vi "Serial Port Read.vi"(7 "stop":bool, 8 "error in (no error)":errorcluster, 9 "Timeout (2000ms)":u32=2000, 10 "Byte Count":u32, 11 "VISA resource name":refnum<visa-resource-name>) -> (0 "error out":errorcluster, 1 "Return Count":u32, 2 "Read Buffer":string, 3 "VISA resource name out":refnum<visa-resource-name>)   [LabVIEW 2009, in "DSO1K.lvlib"]
doc: "Serial port that you set for this vi."
uses:
  <instrlib>/DSO1K/DSO1K.lvlib
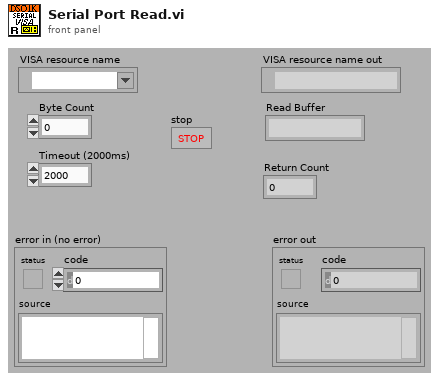
[diagram p1: front panel]
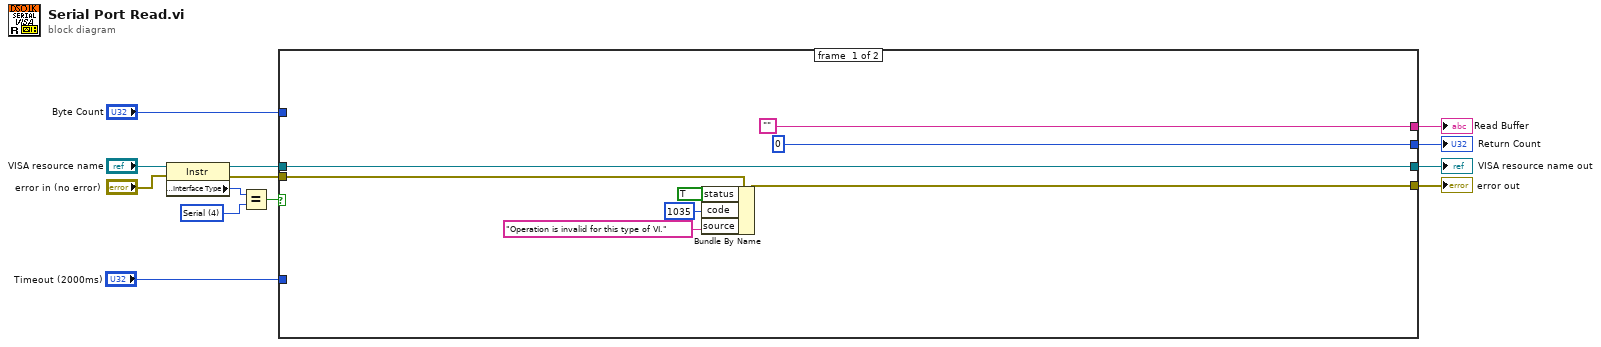
[diagram p0: block diagram]
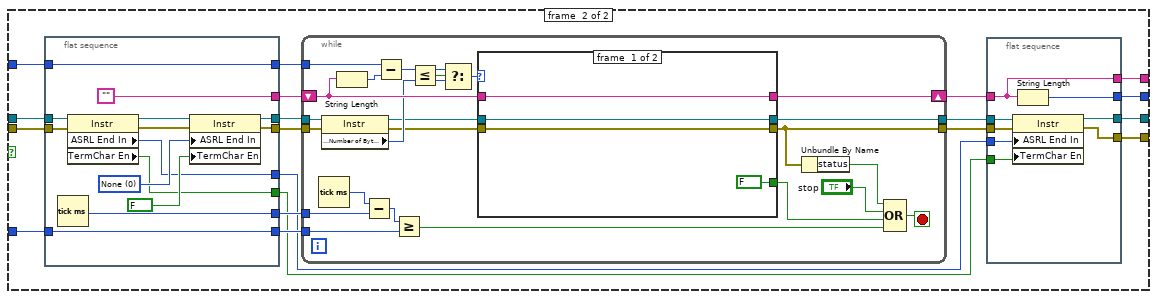
[diagram p2: hidden frame]
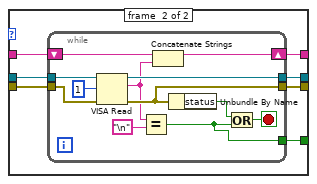
[diagram p3: hidden frame]
diagram:
  w3 = u16 4 items=["GPIB"=1, "VXI"=2, "GPIB-VXI"=3, "Serial"=4, "PXI"=5, "TCPIP"=6, "USB"=7, "FireWire"=9] ("Interface Information:Interface Type")
  n1 = property class="Instr"(reference="VISA resource name", error in="error in (no error)") -> (reference out=w13:refnum<visa-resource-name>, error out=w12:errorcluster, "Interface Information:Interface Type"=w4:u16)
  n2 = Equal?(x=w4, y=w3) -> (x = y?=w2:bool)
  n3 = case shown="True" w2 {
    tunnel: w13 -> [w19 w36]
    tunnel: w12 -> [w18 w35]
    tunnel: ["" w24] -> w6
    tunnel: [w19 w25] -> w9
    tunnel: [w17 w28] -> w8
    tunnel: [u32 0 ("return count") w30] -> w10
    tunnel: "Byte Count" -> [_ w32]
    tunnel: "Timeout (2000ms)" -> [_ w31]
    frame #0 {
      n4 = Bundle By Name(cluster=w18, "status"=TRUE, "code"=1035, "source"="Operation is invalid for this type of VI.") -> (w17:errorcluster)
    }
    frame #1 {
      n5 = flat-sequence {
        tunnel: [w60] -> w40
        tunnel: [w59] -> w39
        tunnel: [w62] -> w38
        tunnel: [""] -> w37
        tunnel: w36 -> [w58]
        tunnel: w35 -> [w57]
        tunnel: [w54] -> w34
        tunnel: [w53] -> w33
        tunnel: w32 -> [w60]
        tunnel: w31 -> [w59]
        tunnel: [w50] -> w23
        tunnel: [w49] -> w22
        frame #0 {
          w52 = u16 0 items=["None", "Last Bit", "TermChar"] ("Serial Settings:End Mode for Reads")
          n6 = Tick Count (ms)() -> (millisecond timer value=w62:u32)
          n7 = property class="Instr"(reference=w58, error in=w57) -> (reference out=w56:refnum<visa-resource-name>, error out=w55:errorcluster, "ASRL End In"=w50:u16, "TermChar En"=w49:bool)
          n8 = property class="Instr"(reference=w56, error in=w55, "ASRL End In"=w52, "TermChar En"=FALSE) -> (reference out=w54:refnum<visa-resource-name>, error out=w53:errorcluster)
        }
      }
      n9 = while {
        shift-right: [w84] -> w29
        shift-left: w37 -> [w79]
        tunnel: [w85] -> w26
        tunnel: [w66] -> w27
        tunnel: w38 -> [w81]
        tunnel: w39 -> [w80]
        tunnel: w34 -> [w78]
        tunnel: w33 -> [w75]
        tunnel: w40 -> [w76]
        stop <- w73 stop-if-true
        n10 = Tick Count (ms)() -> (millisecond timer value=w83:u32)
        n11 = property class="Instr"(reference=w78, error in=w75) -> (reference out=w70:refnum<visa-resource-name>, error out=w69:errorcluster, "Serial Settings:Number of Bytes at Serial Port"=w71:u32)
        n12 = String Length(string=w79) -> (length=w77:i32)
        n13 = Subtract(x=w83, y=w81) -> (x-y=w82:u32)
        n14 = Subtract(x=w76, y=w77) -> (x-y=w72:u32)
        n15 = Greater Or Equal?(x=w82, y=w80) -> (x >= y?=w74:bool)
        n16 = Less Or Equal?(x=w72, y=w71) -> (x <= y?=w68:bool)
        n17 = Select(t=w72, s=w68, f=w71) -> (s? t:f=w67:u32)
        n18 = case shown="1, Default" w67 {
          tunnel: [w88 w96] -> w85
          tunnel: [w89 w91] -> w84
          tunnel: [w87 w95] -> w66
          tunnel: w79 -> [w89 w92]
          tunnel: w70 -> [w88 w94]
          tunnel: w69 -> [w87 w93]
          tunnel: [FALSE w90] -> w63
          frame #0 {
          }
          frame #1 {
            n19 = while {
              tunnel: [w108] -> w96
              tunnel: [w104] -> w95
              tunnel: w94 -> [w107]
              tunnel: w93 -> [w106]
              shift-right: [w98] -> w91
              shift-left: w92 -> [w99]
              tunnel: [w97] -> w90
              stop <- w100 stop-if-true
              n20 = VISA Read(VISA resource name=w107, byte count=u32 1, error in (no error)=w106) -> (VISA resource name out=w108:refnum<visa-resource-name>, read buffer=w103:string, error out=w104:errorcluster)  [unwired: 1 out]
              n21 = Equal?(x=w103, y="\n") -> (x = y?=w97:bool)
              n22 = Concatenate Strings(w99, w103) -> (w98:string)
              n23 = Unbundle By Name(w104) -> ("status"=w101:bool)
              n24 = Or(x=w101, y=w97) -> (x .or. y?=w100:bool)
            }
          }
        }
        n25 = Unbundle By Name(w66) -> ("status"=w65:bool)
        n26 = Compound Arithmetic op=OR(w65, "stop", w63, w74) -> (w73:bool)
      }
      n27 = flat-sequence {
        tunnel: [w48] -> w30
        tunnel: w29 -> [w47]
        tunnel: [w44] -> w28
        tunnel: w27 -> [w43]
        tunnel: [w45] -> w25
        tunnel: w26 -> [w46]
        tunnel: [w47] -> w24
        tunnel: w23 -> [w42]
        tunnel: w22 -> [w41]
        frame #0 {
          n28 = property class="Instr"(reference=w46, error in=w43, "ASRL End In"=w42, "TermChar En"=w41) -> (reference out=w45:refnum<visa-resource-name>, error out=w44:errorcluster)
          n29 = String Length(string=w47) -> (length=w48:i32)
        }
      }
    }
  }
  "VISA resource name out" <- w9
  "error out" <- w8
  "Return Count" <- w10
  "Read Buffer" <- w6
